vi "Get Data Replay Component Properties.vi"(8 "error in (no error)":errorcluster, 9 "Prefix #":i32, 11 "Item Ref in":T1 format="%.0x") -> (0 "error out":errorcluster, 2 "DataReplays":T2[](array[typedef]), 3 "Item Ref out":T1 format="%.0x")   [LabVIEW 2011, in "Engine Sim System Explorer.lvlib"]
uses:
  Engine Sim System Explorer.lvlib
  <vilib>/NI Veristand/Custom Device API/Custom Device Item Ref.ctl
  TypeDefs/DataReplayComp.ctl
  Shared/Engine Simulation Global.vi
  <vilib>/NI Veristand/Custom Device API/Get Item Property (I32).vi
  <vilib>/NI Veristand/Custom Device API/Get Item Property (String).vi
  <vilib>/NI Veristand/Custom Device API/Get Item Property (Variant).vi
  Engine Simulation Shared.lvlib
  <vilib>/NI Veristand/Custom Device API/Custom Device API.lvlib
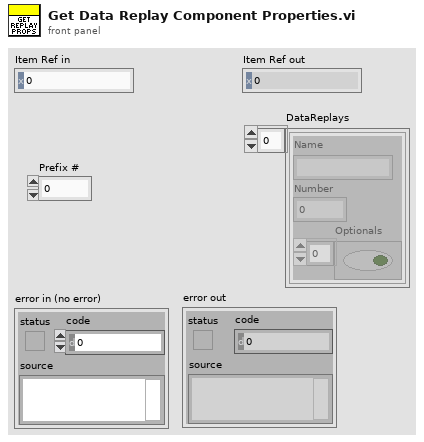
[diagram p1: front panel]
types:
  T1 = typedef "Custom Device API.lvlib/Custom Device Item Ref.ctl" = u64
  T2 = typedef "Engine Sim System Explorer.lvlib/DataReplayComp.ctl" = cluster{"Name":string, "Number":i32, "Optionals":bool[]}
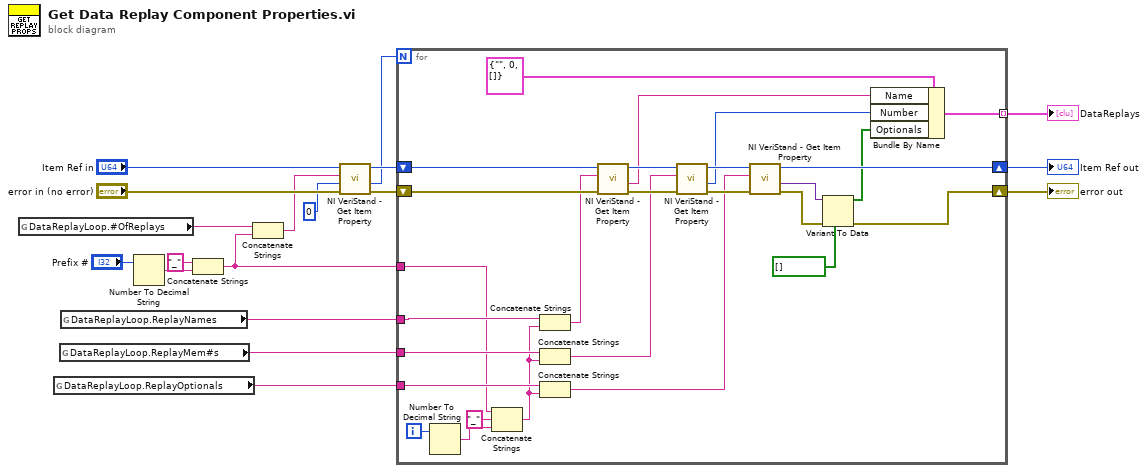
[diagram p0: block diagram]
diagram:
  n1 = global read "Engine Simulation Global.vi" "DataReplayLoop.#OfReplays"() -> (w16:string)
  n2 = global read "Engine Simulation Global.vi" "DataReplayLoop.ReplayOptionals"() -> (w11:string)
  n3 = global read "Engine Simulation Global.vi" "DataReplayLoop.ReplayMem#s"() -> (w12:string)
  n4 = global read "Engine Simulation Global.vi" "DataReplayLoop.ReplayNames"() -> (w13:string)
  n5 = Number To Decimal String(number="Prefix #") -> (decimal integer string=w5:string)  [unwired: 1 in]
  n6 = Concatenate Strings("_" ("string"), w5) -> (w1:string)
  n7 = Concatenate Strings(w16, w1) -> (w2:string)
  n8 = call-poly <vilib>:"NI VeriStand - Get Item Property.vi"("error in (no error)"="error in (no error)", "Default Value"=0, "Property Name"=w2, "Item Ref in"="Item Ref in") -> ("error out"=w15:errorcluster, "Value"=w7:i32, "Item Ref out"=w14:T1)  [unwired: 4 in, 1 out]
  n9 = for {
    N: w7 -> [_]
    shift-right: [w25] -> w10
    shift-left: w15 -> [w38]
    shift-right: [w28] -> w9
    shift-left: w14 -> [w37]
    tunnel: w13 -> [w44]
    tunnel: w12 -> [w41]
    tunnel: w11 -> [w40]
    tunnel: [w20] -> w6 mode=indexing
    tunnel: w1 -> [w19]
    i -> [w45]
    n10 = Number To Decimal String(number=w45) -> (decimal integer string=w43:string)  [unwired: 1 in]
    n11 = Concatenate Strings(w19, "_" ("string"), w43) -> (w39:string)
    n12 = Concatenate Strings(w44, w39) -> (w36:string)
    n13 = Concatenate Strings(w41, w39) -> (w33:string)
    n14 = Concatenate Strings(w40, w39) -> (w30:string)
    n15 = call-poly <vilib>:"NI VeriStand - Get Item Property.vi"("error in (no error)"=w38, "Property Name"=w36, "Item Ref in"=w37) -> ("error out"=w35:errorcluster, "Value"=w26:string, "Item Ref out"=w34:T1)  [unwired: 5 in, 1 out]
    n16 = call-poly <vilib>:"NI VeriStand - Get Item Property.vi"("error in (no error)"=w35, "Property Name"=w33, "Item Ref in"=w34) -> ("error out"=w32:errorcluster, "Value"=w22:i32, "Item Ref out"=w31:T1)  [unwired: 5 in, 1 out]
    n17 = call-poly <vilib>:"NI VeriStand - Get Item Property.vi"("error in (no error)"=w32, "Property Name"=w30, "Item Ref in"=w31) -> ("error out"=w29:errorcluster, "Value"=w24:variant, "Item Ref out"=w28:T1)  [unwired: 5 in, 1 out]
    n18 = Variant To Data(error in=w29, type=bool[] [], Variant=w24) -> (data=w21:bool[], error out=w25:errorcluster)
    n19 = Bundle By Name(cluster=T2 {"Name"="", "Number"=0, "Optionals"=[]} ("input cluster"), "Name"=w26, "Number"=w22, "Optionals"=w21) -> (w20:T2)
  }
  "error out" <- w10
  "DataReplays" <- w6
  "Item Ref out" <- w9
